vi "calculate_drivable_paths.vi"(11 "allowed proximity squared":i16=400) -> ()   [LabVIEW 2009]
uses:
  <vilib>/rvi/DataTransferAndStorage/Container/XNode/niFpgaContainer.xnode
  <vilib>/rvi/FIFO/Fifo_Resource/nirvififoUniquifyingName.vi
  athena FPGA globals.vi
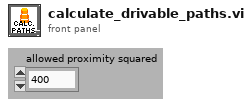
[diagram p1: front panel]
types:
  T1 = enum16{"confirm check sum", "check status byte", "read measured values", "confirm measurement", "confirm command", "read message length", "read address", "wait for \"02\""}
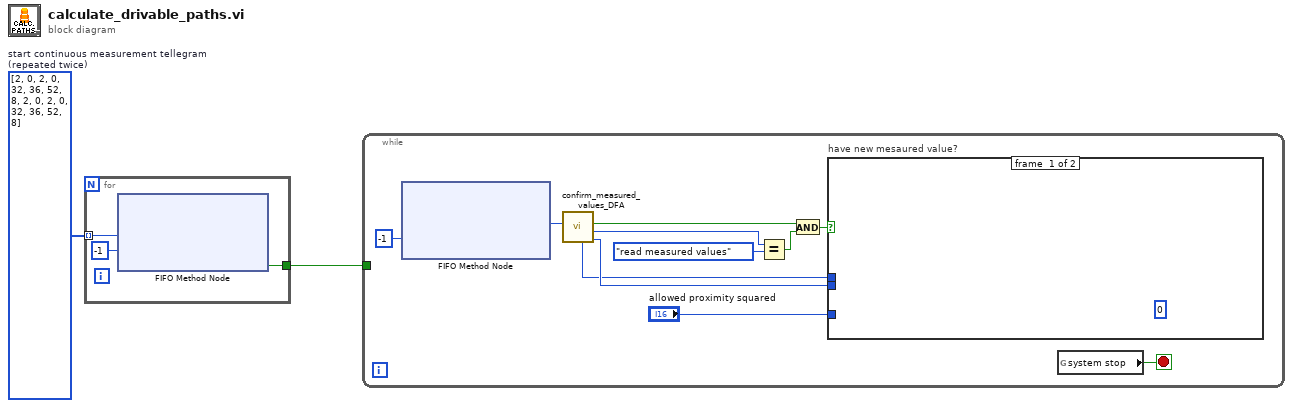
[diagram p0: block diagram]
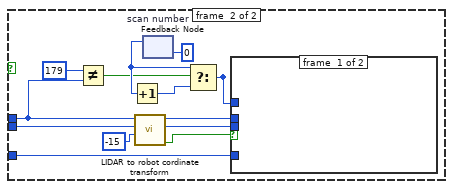
[diagram p2: hidden frame]
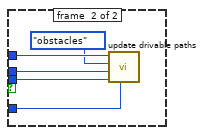
[diagram p3: hidden frame]
diagram:
  w1 = u8[] [2, 0, 2, 0, 32, 36, 52, 8, 2, 0, 2, 0, 32, 36, 52, 8]  # start continuous measurement tellegram (repeated twice)
  n1 = for {
    tunnel: w1 -> [w5] mode=indexing
    tunnel: [w3] -> w2
    n2 = xnode ("FIFO Method Node")("Element"=w5, "Timeout"=-1) -> ("Timed Out?"=w3:bool)  [unwired: 1 in, 1 out]
  }
  n3 = while {
    tunnel: w2 -> [_]
    stop <- w55 stop-if-true
    n4 = xnode ("FIFO Method Node")("Timeout"=-1) -> ("Element"=w64:u8)  [unwired: 1 in, 2 out]
    n5 = call "confirm_measured_values_DFA.vi"("LIDAR raw data"=w64) -> ("last measured value"=w63:u16, "parser state"=w62:T1, "new value?"=w61:bool, "angle"=w57:u8)  [unwired: 7 in]
    n6 = Equal?(x=w62, y=T1."read measured values" ("parser state")) -> (x = y?=w58:bool)
    n7 = And(x=w61, y=w58) -> (x .and. y?=w60:bool)
    n8 = case "have new mesaured value?" shown="True" w60 {
      tunnel: w63 -> [_ w125]
      tunnel: w57 -> [_ w118]
      tunnel: "allowed proximity squared" -> [_ w113]
      frame #0 {
        (unwired) u8 0 ("y")
      }
      frame #1 {
        n9 = Not Equal?(x=u8 179, y=w118) -> (x != y?=w119:bool)
        n10 = call "LIDAR to robot cordinate transform.vi"("Lidar Vertical Position"=i8 -15, "Lidar Distance"=w125, "Lidar Scan Angle"=w118) -> ("Is object?"=w122:bool, "Robot Y"=w123:i16, "Lidar X = Robot X"=w124:i16)  [unwired: 3 in, 3 out]
        n11 = feedback #1 "scan number"(u8 0 ("y")) -> (w121:u8)
        n12 = Increment(x=w121) -> (x+1=w120:u8)
        n13 = Select(t=w121, s=w119, f=w120) -> (s? t:f=w116:u8)
        n14 = case shown="True" w122 {
          tunnel: w124 -> [_ w130]
          tunnel: w123 -> [_ w129]
          tunnel: w116 -> [_ w128]
          tunnel: w113 -> [_ w126]
          frame #0 {
          }
          frame #1 {
            n15 = call "update drivable paths.vi"("allowed proximity squared"=w126, "Robot Y"=w129, "Robot X"=w130, "update lines or objects"=enum16{"lines", "obstacles"}."obstacles", "Scan Number"=w128) -> ()  [unwired: 7 in]
          }
        }
      }
    }
    n16 = global read "athena FPGA globals.vi" "system stop"() -> (w55:bool)
  }
